vi "ExCore1_01.vi"(4 "error in":errorcluster, 5 "B":dbl, 7 "A":dbl) -> (0 "error out":errorcluster, 1 "D":dbl, 3 "S":dbl)   [LabVIEW 2021]
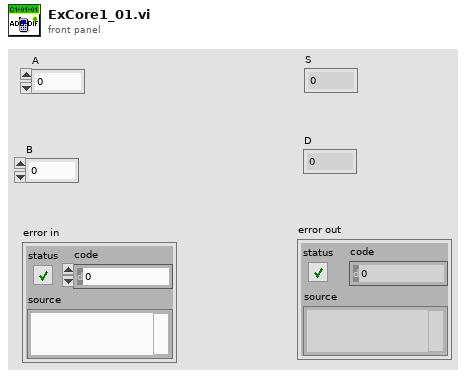
[diagram p1: front panel]
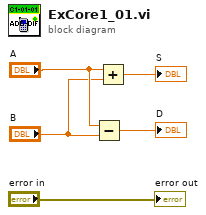
[diagram p0: block diagram]
diagram:
  n1 = Subtract(x="A", y="B") -> (x-y=→"D":dbl)
  n2 = Add(x="A", y="B") -> (x+y=→"S":dbl)
  "error out" <- "error in"
